vi "selectPathToOpen.vi"(8 "error in (no error)":errorcluster, 11 "ImageStreamViewer in":refnum<class "ImageStreamViewer.lvclass">) -> (0 "error out":errorcluster, 1 "selected path":path, 2 "notSelected?":bool, 3 "ImageStreamViewer out":refnum<class "ImageStreamViewer.lvclass">)   [LabVIEW 2011, in "Views.lvlib" / "Camera.lvlib" / "ImageStreamViewer.lvclass"]
uses:
  ImageStreamViewer.lvclass
  Tools/Filing/FileSystem/FileSystem.lvclass
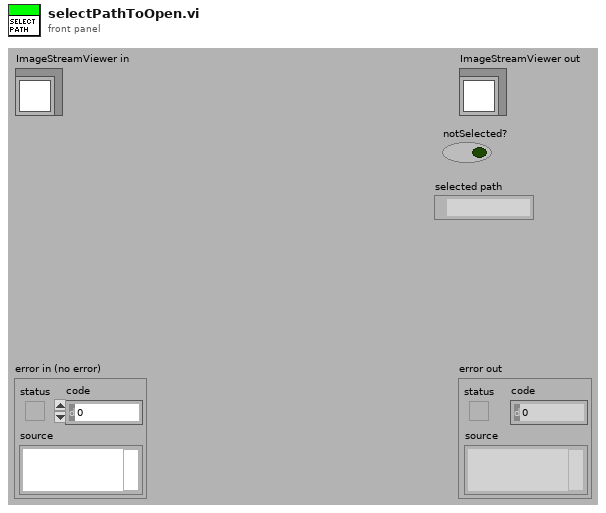
[diagram p1: front panel]
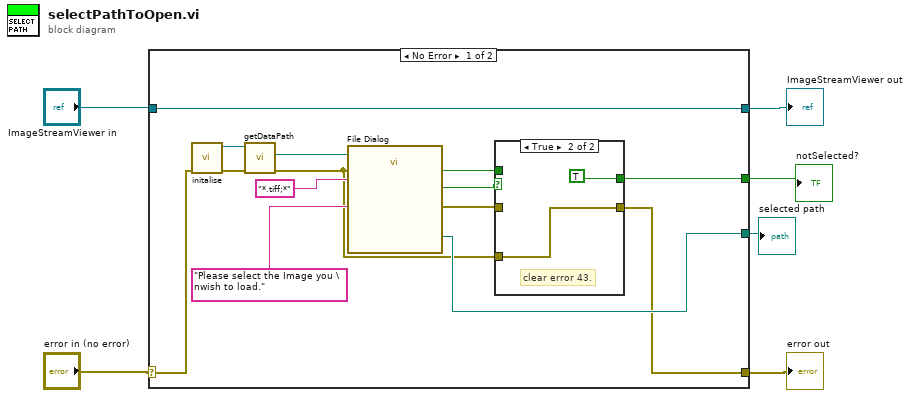
[diagram p0: block diagram]
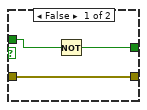
[diagram p2: hidden frame]
diagram:
  n1 = case shown="No Error" "error in (no error)" {
    selector: "error in (no error)" -> [w8 w27]
    tunnel: [w9 w27] -> w4
    tunnel: [w20 w26] -> w5
    tunnel: "ImageStreamViewer in" -> [w20 w26]
    tunnel: [w12 _] -> w2
    tunnel: [w14 _] -> w1
    frame No Error {
      n2 = call "initalise.vi"("error in (no error)"=w8) -> ("error out"=w17:errorcluster, "FileSystem out"=w18:refnum<class "FileSystem.lvclass">)  [unwired: 9 in]
      n3 = call-dynamic "getDataPath.vi"("error in (no error)"=w17, "FileSystem.lvclass in"=w18) -> ("error out"=w7:errorcluster, "DataPath"=w19:path)  [unwired: 7 in, 1 out]
      n4 = call "File Dialog"("start path"=w19, "prompt"="Please select the Image you \nwish to load.", "error in"=w7, "pattern (all files)"="*.tiff;*") -> ("selected path"=w14:path, "exists"=w11:bool, "cancelled"=w13:bool, "error out"=w10:errorcluster)  [unwired: 8 in]
      n5 = case shown="True" w13 {
        tunnel: [w22 TRUE] -> w12
        tunnel: w11 -> [w23 _]
        tunnel: w10 -> [w21 _]
        tunnel: [w21 w24] -> w9
        tunnel: w7 -> [_ w24]
        frame False {
          n6 = Not(x=w23) -> (.not. x?=w22:bool)
        }
        frame True {
          # "clear error 43."
        }
      }
    }
    frame Error {
    }
  }
  "error out" <- w4
  "ImageStreamViewer out" <- w5
  "notSelected?" <- w2
  "selected path" <- w1
